vi "button press.vi"(11 "button IN":bool) -> (3 "Button Pressed?":bool)   [LabVIEW 2023]
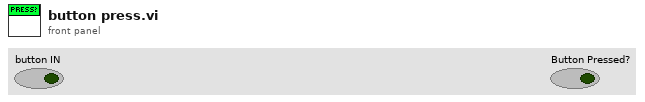
[diagram p1: front panel]
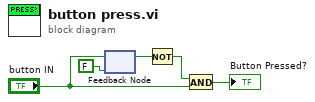
[diagram p0: block diagram]
diagram:
  n1 = feedback-in #1("button IN") -> ()
  n2 = feedback #1(FALSE ("button IN")) -> (w5:bool)
  n3 = Not(x=w5) -> (.not. x?=w3:bool)
  n4 = And(x=w3, y="button IN") -> (x .and. y?=→"Button Pressed?":bool)
